vi "Universal B-IV-V.vi"() -> ()   [LabVIEW 2023]
uses:
  <vilib>/Utility/file.llb/Write Delimited Spreadsheet (DBL).vi
panel:
  out "Waveform Graph 2":dbl[](graph)
  out "error out":errorcluster
  out "Current Field":dbl
  out "Waveform Graph":dbl[](graph)
  in  "Tab Control":enum32{"Log", "Module Choose", "Range"}(tab)=enum."Range"
  in  "File Name":string="test"
  in  "base path":path=path "C:/Users/gyue/Box/Guang Yue uiuc research box folder/data/Contour plot"
  out "Generated File name":string
  in  "Book number":i32=545
  in  "Channel 2":bool=TRUE
  in  "Choose Data Channel 2":enum32{"None", "SR760 FFT"}(tab)=enum."SR760 FFT"
  in  "GPIB address 2":string="10"
  in  "Channel 1":bool=TRUE
  in  "Choose Data Channel 1":enum32{"None", "cRIO IV", "SR760 FFT"}(tab)=enum."cRIO IV"
  in  "GPIB address":string="10"
  in  "Magnet Control":enum32{"None", "Elsa 5T", "Keithley 2400"}(tab)=enum."Elsa 5T"
  in  "Field Rate mT per sec":dbl=0.1 format="%#_13g"
  in  "Field Origin":dbl format="%#_13g"
  in  "Field step":dbl=0.1 format="%#_13g"
  in  "Field Radius":dbl=1.0 format="%#_13g"
  in  "Ramp up first T":bool=TRUE
  in  "Ramp type":string(combo)="Origin is Boundary"
  in  "Delay Time s":dbl=1.0 caption="Delay Time (s)"
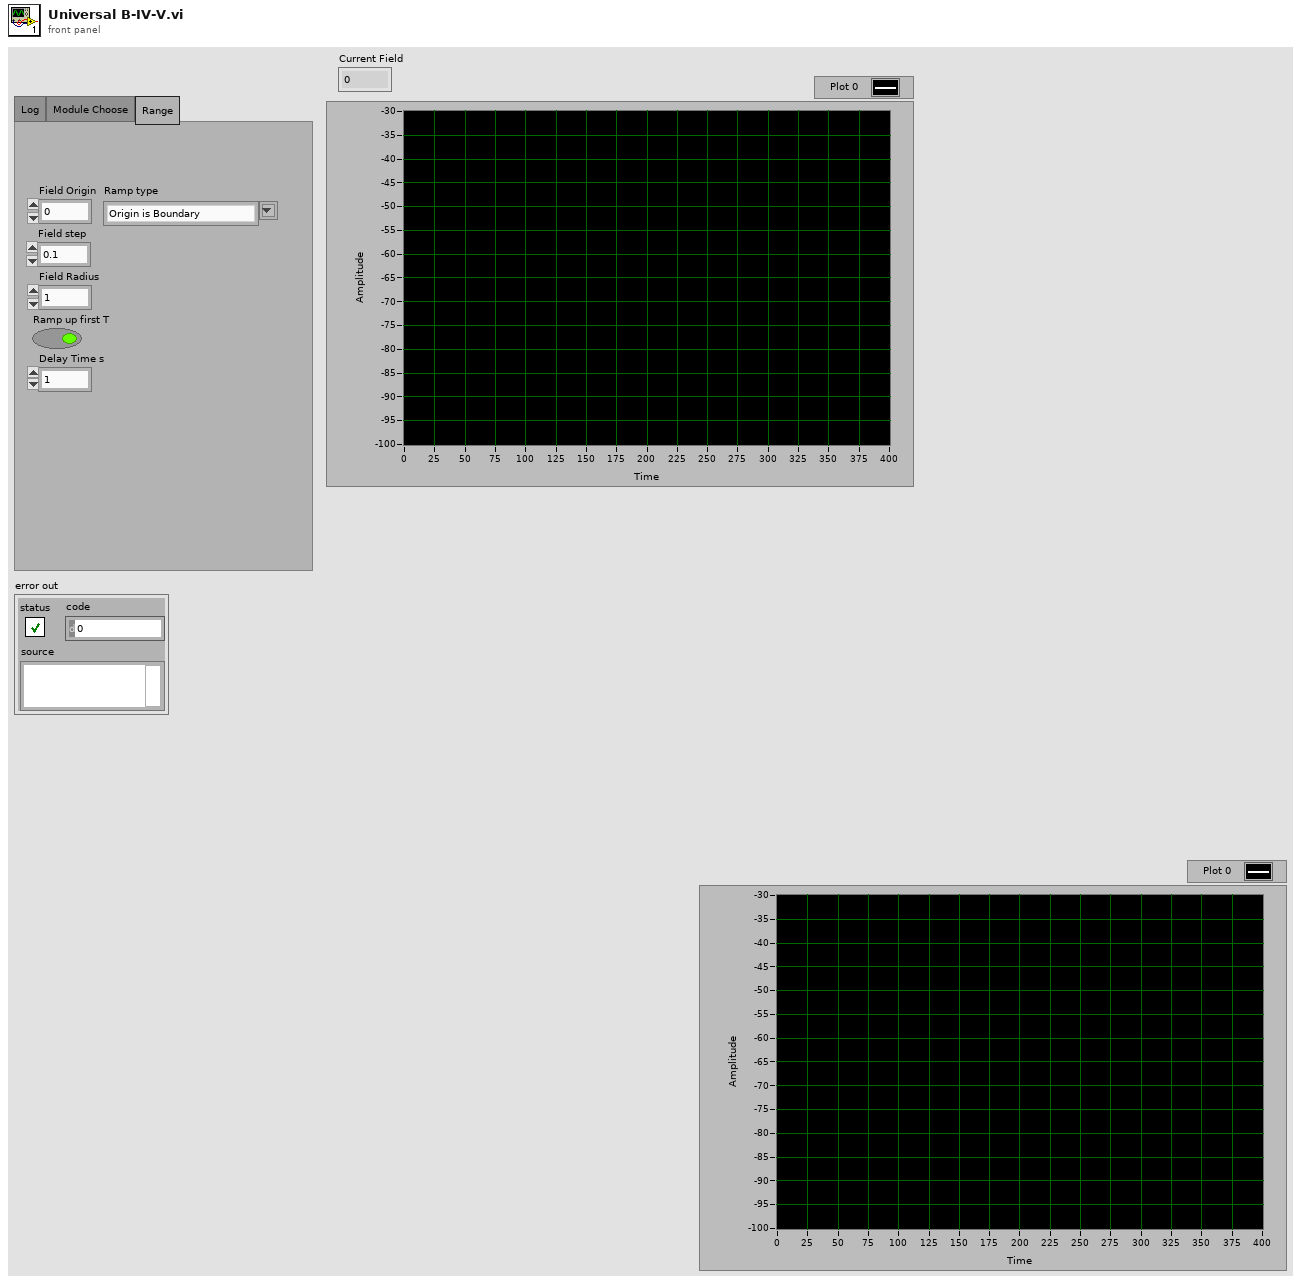
[diagram p1: front panel]
types:
  T1 = cluster{"error":bool, "code":i32, "source":string}
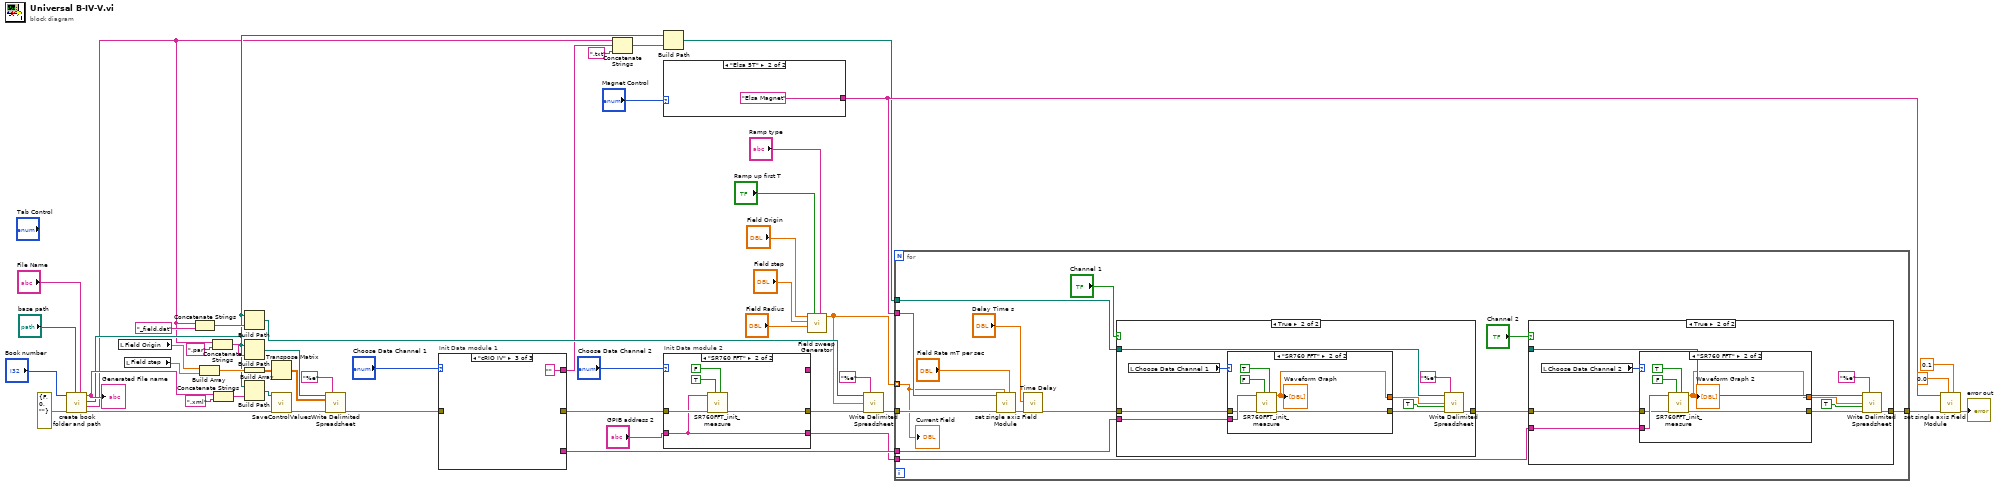
[diagram p0: block diagram]
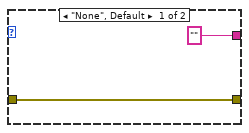
[diagram p2: hidden frame]
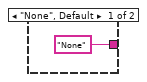
[diagram p3: hidden frame]
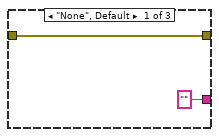
[diagram p4: hidden frame]
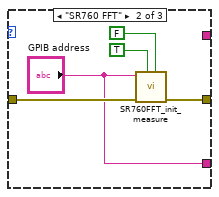
[diagram p5: hidden frame]
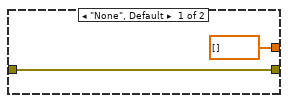
[diagram p7: hidden frame]
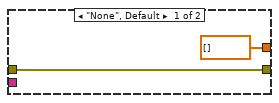
[diagram p9: hidden frame]
diagram:
  n1 = call "create book folder and path.vi"("File Name"="File Name", "base path"="base path", "error in"=errorcluster {"status"=FALSE, "code"=0, "source"=""}, "Book number"="Book number") -> ("error out"=w1:errorcluster, "book name"=w2:string, "appended path"=w3:path, "timed File name"=w5:string)  [unwired: 4 in]
  "Generated File name" <- w5
  n2 = local read "Field Origin"() -> (w28:dbl)
  n3 = local read "Field step"() -> (w27:dbl)
  n4 = Concatenate Strings(w2, "_field.dat" ("string")) -> (w30:string)
  n5 = Build Array(w28, w27) -> (w26:dbl[])
  n6 = Concatenate Strings(w2, ".par" ("string")) -> (w32:string)
  n7 = Concatenate Strings(w5, ".xml" ("string")) -> (w50:string)
  n8 = Build Path(base path=w3, name or relative path=w30) -> (appended path=w18:path)
  n9 = Build Path(base path=w3, name or relative path=w32) -> (appended path=w21:path)
  n10 = Build Array(w26) -> (w25:dbl[][])
  n11 = Build Path(base path=w3, name or relative path=w50) -> (appended path=w49:path)
  n12 = Transpose Matrix(1:w25) -> (0:w24:dbl[][])
  n13 = call "SaveControlValues.vi"("XML File Path"=w49, "error in (no error)"=w1) -> ("error out"=w22:errorcluster)  [unwired: 8 in]
  n14 = call-poly <vilib>:"Write Delimited Spreadsheet.vi"("file path (dialog if empty)"=w21, "format (%.3f)"="%e", "2D data"=w24, "error in (no error)"=w22) -> ("error out"=w20:errorcluster)  [unwired: 10 in, 1 out]
  n15 = case "Init Data module 1" shown="\"cRIO IV\"" "Choose Data Channel 1" {
    tunnel: w20 -> [w52 w55 _]
    tunnel: [w52 w54 _] -> w15
    tunnel: ["" ("GPIB address") "GPIB address" _] -> w38
    tunnel: [_ _ ""] -> w11
    frame "None", Default {
    }
    frame "SR760 FFT" {
      n16 = call "SR760FFT_init_measure.vi"("Measure"=FALSE, "Init"=TRUE, "error in"=w55, "GPIB address"="GPIB address") -> ("error out"=w54:T1)  [unwired: 6 in, 1 out]
    }
    frame "cRIO IV" {
    }
  }
  n17 = Concatenate Strings(w2, w11, ".txt" ("string")) -> (w47:string)
  n18 = Build Path(base path=w3, name or relative path=w47) -> (appended path=w29:path)
  n19 = case shown="\"Elsa 5T\"" "Magnet Control" {
    tunnel: ["None" "Elsa Magnet"] -> w36
    frame "None", Default {
    }
    frame "Elsa 5T" {
    }
  }
  n20 = case "Init Data module 2" shown="\"SR760 FFT\"" "Choose Data Channel 2" {
    tunnel: w15 -> [w62 w65]
    tunnel: [w62 w64] -> w13
    tunnel: ["" ("GPIB address") _] -> _
    tunnel: "GPIB address 2" -> [_ w63]
    tunnel: [_ w63] -> w9
    frame "None", Default {
    }
    frame "SR760 FFT" {
      n21 = call "SR760FFT_init_measure.vi"("Measure"=FALSE, "Init"=TRUE, "error in"=w65, "GPIB address"=w63) -> ("error out"=w64:T1)  [unwired: 6 in, 1 out]
    }
  }
  n22 = call "Field sweep Generator.vi"("Ramp type"="Ramp type", "Ramp up first T"="Ramp up first T", "Field Radius"="Field Radius", "Field step"="Field step", "Field Origin"="Field Origin") -> ("output array"=w17:dbl[])  [unwired: 6 in]
  n23 = call-poly <vilib>:"Write Delimited Spreadsheet.vi"("file path (dialog if empty)"=w18, "format (%.3f)"="%e", "1D data"=w17, "error in (no error)"=w13) -> ("error out"=w16:errorcluster)  [unwired: 10 in, 1 out]
  n24 = for {
    tunnel: w17 -> [w79] mode=indexing
    tunnel: w16 -> [w81]
    tunnel: w36 -> [w80]
    tunnel: w38 -> [w75]
    tunnel: [w69] -> w37
    tunnel: w29 -> [w72]
    tunnel: w9 -> [w68]
    n25 = call "set single axis Field Module.vi"("Field Rate mT per sec"="Field Rate mT per sec", "Field Target mT"=w79, "error in (no error)"=w81, "Device Select"=w80) -> ("error out"=w76:errorcluster)  [unwired: 7 in]
    n26 = call "Time Delay"("error in (no error)"=w76, "Delay Time (s)"="Delay Time s") -> ("error out"=w74:errorcluster)  [unwired: 9 in]
    n27 = case shown="True" "Channel 1" {
      tunnel: w75 -> [_ w108]
      tunnel: w74 -> [w100 w107]
      tunnel: w72 -> [_ w106]
      tunnel: [w100 w101] -> w70
      frame False {
      }
      frame True {
        n28 = local read "Choose Data Channel 1"() -> (w109:enum32{"None", "cRIO IV", "SR760 FFT"})
        n29 = case shown="\"SR760 FFT\"" w109 {
          tunnel: w108 -> [_ w115]
          tunnel: w107 -> [w111 w114]
          tunnel: [w111 w113] -> w102
          tunnel: [dbl[] [] ("Array") w112] -> w104
          frame "None", Default {
          }
          frame "SR760 FFT" {
            n30 = call "SR760FFT_init_measure.vi"("Measure"=TRUE, "Init"=FALSE, "error in"=w114, "GPIB address"=w115) -> ("error out"=w113:T1, "Array"=w112:dbl[])  [unwired: 6 in]
            "Waveform Graph" <- w112
          }
        }
        n31 = call-poly <vilib>:"Write Delimited Spreadsheet.vi"("file path (dialog if empty)"=w106, "format (%.3f)"="%e", "1D data"=w104, "append to file? (new file:F)"=TRUE, "error in (no error)"=w102) -> ("error out"=w101:errorcluster)  [unwired: 9 in, 1 out]
      }
    }
    n32 = case shown="True" "Channel 2" {
      tunnel: w68 -> [_ w90]
      tunnel: w70 -> [w82 w89]
      tunnel: _ -> [_ w88]
      tunnel: [w82 w83] -> w69
      frame False {
      }
      frame True {
        n33 = local read "Choose Data Channel 2"() -> (w91:enum32{"None", "SR760 FFT"})
        n34 = case shown="\"SR760 FFT\"" w91 {
          tunnel: w90 -> [_ w97]
          tunnel: w89 -> [w93 w96]
          tunnel: [w93 w95] -> w84
          tunnel: [dbl[] [] ("Array") w94] -> w86
          frame "None", Default {
          }
          frame "SR760 FFT" {
            n35 = call "SR760FFT_init_measure.vi"("Measure"=TRUE, "Init"=FALSE, "error in"=w96, "GPIB address"=w97) -> ("error out"=w95:T1, "Array"=w94:dbl[])  [unwired: 6 in]
            "Waveform Graph 2" <- w94
          }
        }
        n36 = call-poly <vilib>:"Write Delimited Spreadsheet.vi"("file path (dialog if empty)"=w88, "format (%.3f)"="%e", "1D data"=w86, "append to file? (new file:F)"=TRUE, "error in (no error)"=w84) -> ("error out"=w83:errorcluster)  [unwired: 9 in, 1 out]
      }
    }
    "Current Field" <- w79
  }
  n37 = call "set single axis Field Module.vi"("Field Rate mT per sec"=0.1, "Field Target mT"=0.0, "error in (no error)"=w37, "Device Select"=w36) -> ("error out"=→"error out":errorcluster)  [unwired: 7 in]
